vi "getSuperKControls.vi"(6 "error in (no error)":errorcluster, 9 "COMport":string="COM6") -> (0 "error out":errorcluster, 2 "output cluster":T1)   [LabVIEW 2015]
panel:
  out "internalPulseFreqLimitHz":u32
  out "watchdogIntervalSec":u8
  out "burstPulses":u16
  out "internalPulseFreqHz":u16
  out "trigMode":u8
  out "displayBacklightPercent":u8
  out "trigLevelSetpointmV":u16
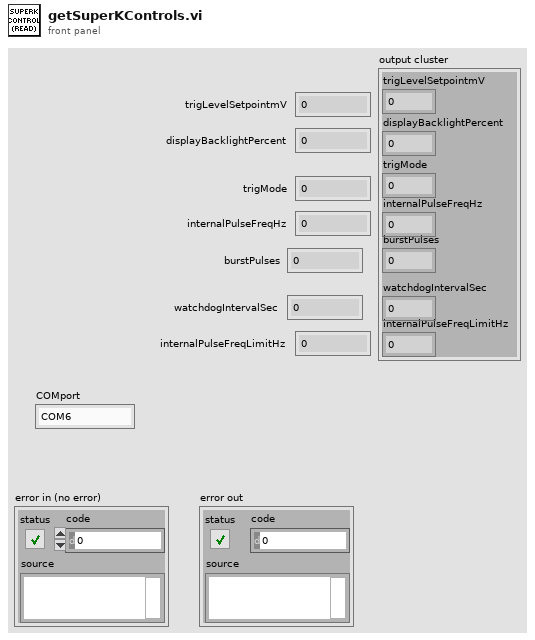
[diagram p1: front panel]
types:
  T1 = cluster{"trigLevelSetpointmV":u16, "displayBacklightPercent":u8, "trigMode":u8, "internalPulseFreqHz":u16, "burstPulses":u16, "watchdogIntervalSec":u8, "internalPulseFreqLimitHz":u32}
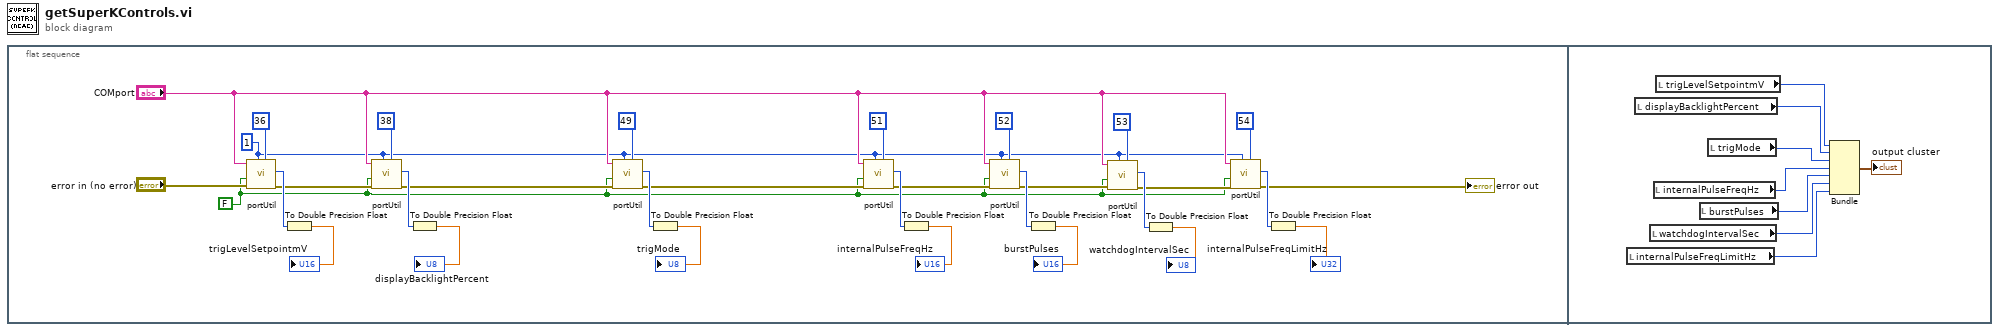
[diagram p0: block diagram]
diagram:
  n1 = flat-sequence {
    frame #0 {
      w9 = FALSE ("WriteNotRead")
      w10 = u8 1 ("Destination")
      n2 = call "portUtil.vi"("Register"=u8 36, "Destination"=w10, "error in (no error)"="error in (no error)", "WriteNotRead"=w9, "COMport"="COMport") -> ("error out"=w28:errorcluster, "Long"=w31:i32)  [unwired: 4 in, 1 out]
      n3 = To Double Precision Float(number=w31) -> (double precision float=→"trigLevelSetpointmV":dbl)
      n4 = call "portUtil.vi"("Register"=u8 38, "Destination"=w10, "error in (no error)"=w28, "WriteNotRead"=w9, "COMport"="COMport") -> ("error out"=w12:errorcluster, "Long"=w29:i32)  [unwired: 4 in, 1 out]
      n5 = To Double Precision Float(number=w29) -> (double precision float=→"displayBacklightPercent":dbl)
      n6 = call "portUtil.vi"("Register"=u8 49, "Destination"=w10, "error in (no error)"=w12, "WriteNotRead"=w9, "COMport"="COMport") -> ("error out"=w11:errorcluster, "Long"=w25:i32)  [unwired: 4 in, 1 out]
      n7 = To Double Precision Float(number=w25) -> (double precision float=→"trigMode":dbl)
      n8 = call "portUtil.vi"("Register"=u8 51, "Destination"=w10, "error in (no error)"=w11, "WriteNotRead"=w9, "COMport"="COMport") -> ("error out"=w16:errorcluster, "Long"=w23:i32)  [unwired: 4 in, 1 out]
      n9 = To Double Precision Float(number=w23) -> (double precision float=→"internalPulseFreqHz":dbl)
      n10 = call "portUtil.vi"("Register"=u8 52, "Destination"=w10, "error in (no error)"=w16, "WriteNotRead"=w9, "COMport"="COMport") -> ("error out"=w15:errorcluster, "Long"=w21:i32)  [unwired: 4 in, 1 out]
      n11 = To Double Precision Float(number=w21) -> (double precision float=→"burstPulses":dbl)
      n12 = call "portUtil.vi"("Register"=u8 53, "Destination"=w10, "error in (no error)"=w15, "WriteNotRead"=w9, "COMport"="COMport") -> ("error out"=w14:errorcluster, "Long"=w19:i32)  [unwired: 4 in, 1 out]
      n13 = To Double Precision Float(number=w19) -> (double precision float=→"watchdogIntervalSec":dbl)
      n14 = call "portUtil.vi"("Register"=u8 54, "Destination"=w10, "error in (no error)"=w14, "WriteNotRead"=w9, "COMport"="COMport") -> ("error out"=→"error out":errorcluster, "Long"=w17:i32)  [unwired: 4 in, 1 out]
      n15 = To Double Precision Float(number=w17) -> (double precision float=→"internalPulseFreqLimitHz":dbl)
    }
    frame #1 {
      n16 = local read "internalPulseFreqLimitHz"() -> (w40:u32)
      n17 = local read "displayBacklightPercent"() -> (w35:u8)
      n18 = local read "watchdogIntervalSec"() -> (w39:u8)
      n19 = local read "internalPulseFreqHz"() -> (w37:u16)
      n20 = local read "trigLevelSetpointmV"() -> (w34:u16)
      n21 = local read "burstPulses"() -> (w38:u16)
      n22 = local read "trigMode"() -> (w36:u8)
      n23 = Bundle("trigLevelSetpointmV"=w34, "displayBacklightPercent"=w35, "trigMode"=w36, "internalPulseFreqHz"=w37, "burstPulses"=w38, "watchdogIntervalSec"=w39, "internalPulseFreqLimitHz"=w40) -> (→"output cluster":T1)  [unwired: 1 in]
    }
  }
